vi "sub vi - cycle&temp fail v7.vi"(0 "Amps Lo?":bool, 2 "Input Cluster":T1, 3 "SELECT":T2(ring), 4 "Amps Hi?":bool, 5 "Result In":bool) -> (15 "(FAIL) out":cluster{"FAIL LO":dbl, "FAIL HI":dbl}, 16 "(DISP) out":T3, 17 "T-RISE":cluster{"T-RISE (L)":dbl, "T-RISE (N)":dbl}, 18 "Result Out":bool, 19 "file error":errorcluster)   [LabVIEW 2017]
uses:
  Global display 3.vi
  Global 1.vi
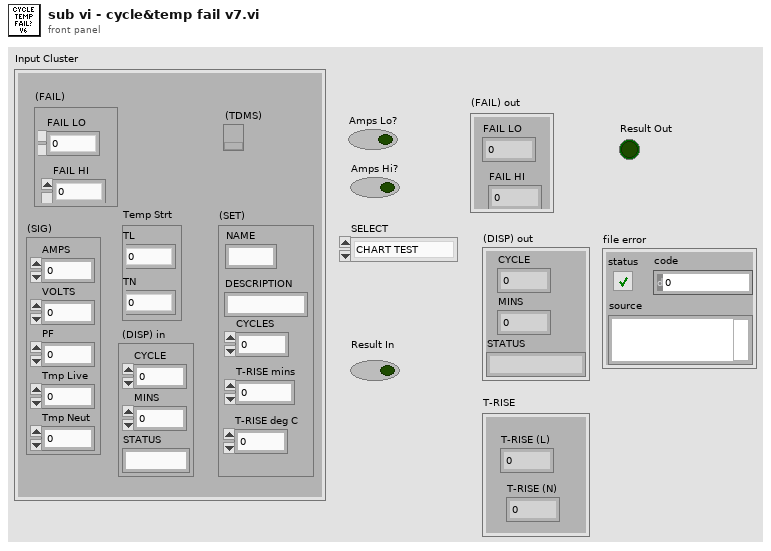
[diagram p1: front panel]
types:
  T1 = cluster{"(FAIL)":cluster{"FAIL LO":dbl, "FAIL HI":dbl}, "(SIG)":cluster{"AMPS":dbl, "VOLTS":dbl, "PF":dbl, "Tmp Live":dbl, "Tmp Neut":dbl}, "Temp Strt":cluster{"TL":dbl, "TN":dbl}, " (DISP) in":cluster{"CYCLE":dbl, "MINS":dbl, "STATUS":string}, "(SET)":cluster{"NAME":string, "DESCRIPTION":string, "CYCLES":dbl, "T-RISE mins":dbl, "T-RISE deg C":dbl}, "(TDMS)":refnum<k34>}
  T2 = enum32{"CHART TEST", "CYCLE TEST", "T-RISE TEST"}
  T3 = cluster{"CYCLE":dbl, "MINS":dbl, "STATUS":string}
  T4 = cluster{"AMPS":dbl, "VOLTS":dbl, "PF":dbl, "Tmp Live":dbl, "Tmp Neut":dbl}
  T5 = cluster{"NAME":string, "DESCRIPTION":string, "CYCLES":dbl, "T-RISE mins":dbl, "T-RISE deg C":dbl}
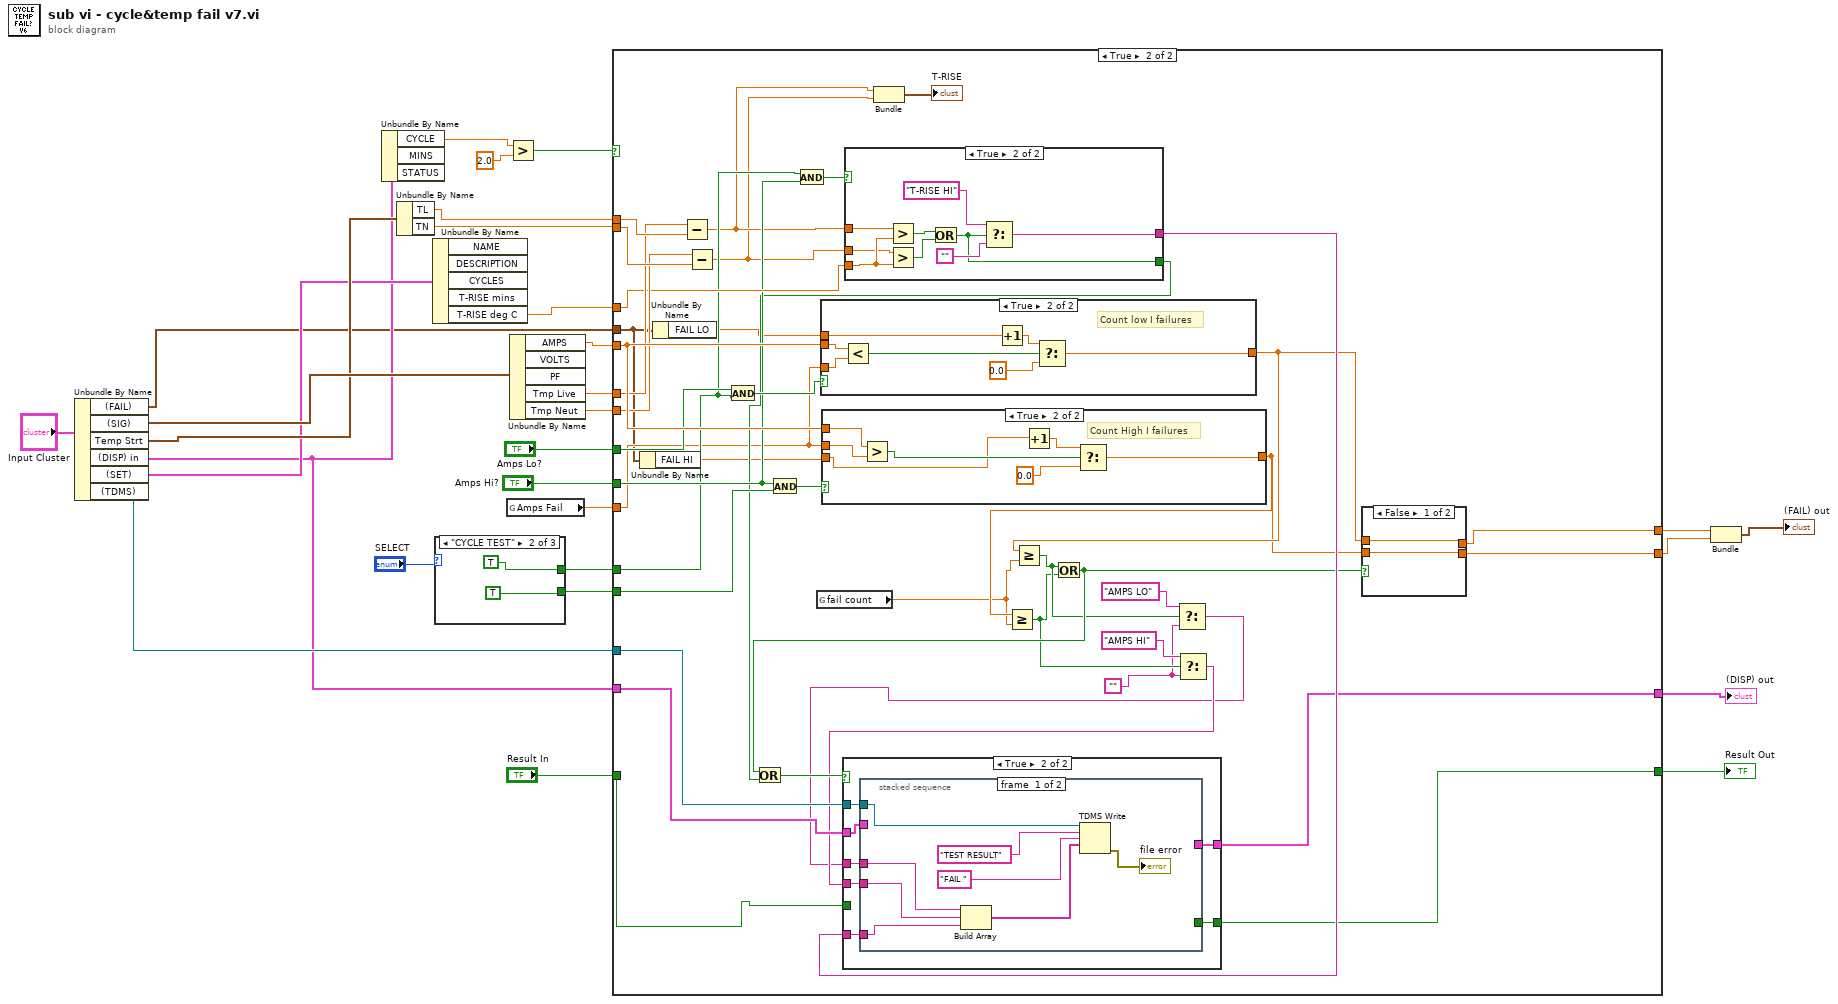
[diagram p0: block diagram]
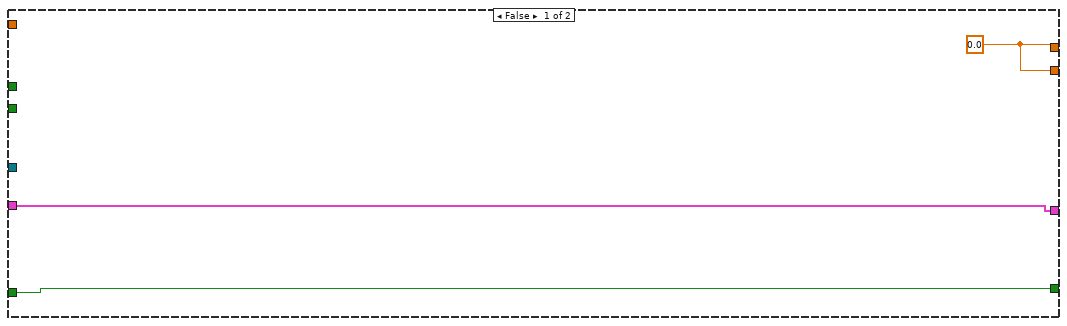
[diagram p2: hidden frame]
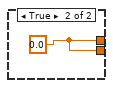
[diagram p3: hidden frame]
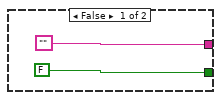
[diagram p4: hidden frame]
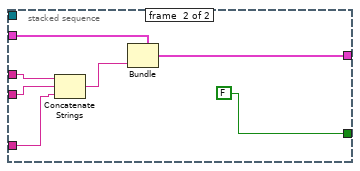
[diagram p6: hidden frame]
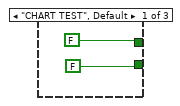
[diagram p9: hidden frame]
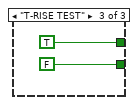
[diagram p10: hidden frame]
diagram:
  n1 = Unbundle By Name("Input Cluster") -> ("(FAIL)"=w1:cluster{"FAIL LO":dbl, "FAIL HI":dbl}, "(SIG)"=w16:T4, "Temp Strt"=w15:cluster{"TL":dbl, "TN":dbl}, "(DISP) in"=w6:T3, "(SET)"=w14:T5, "(TDMS)"=w13:refnum<k34>)
  n2 = Unbundle By Name(w6) -> ("CYCLE"=w5:dbl)  [unwired: 2 out]
  n3 = Unbundle By Name(w15) -> ("TL"=w3:dbl, "TN"=w2:dbl)
  n4 = Unbundle By Name(w14) -> ("T-RISE deg C"=w24:dbl)  [unwired: 4 out]
  n5 = case shown="\"CYCLE TEST\"" "SELECT" {
    tunnel: [FALSE TRUE TRUE] -> w20
    tunnel: [FALSE TRUE FALSE] -> w23
    frame "CHART TEST", Default {
    }
    frame "CYCLE TEST" {
    }
    frame "T-RISE TEST" {
    }
  }
  n6 = global read "Global display 3.vi" "Amps Fail"() -> (w4:dbl)
  n7 = Greater?(x=w5, y=2.0) -> (0:w18:bool)
  n8 = Unbundle By Name(w16) -> ("AMPS"=w27:dbl, "Tmp Live"=w26:dbl, "Tmp Neut"=w25:dbl)  [unwired: 2 out]
  n9 = case shown="True" w18 {
    tunnel: w27 -> [_ w78]
    tunnel: w13 -> [_ w77]
    tunnel: w6 -> [w36 w76]
    tunnel: w3 -> [_ w75]
    tunnel: w2 -> [_ w74]
    tunnel: w26 -> [_ w73]
    tunnel: w25 -> [_ w72]
    tunnel: w24 -> [_ w71]
    tunnel: w23 -> [_ w68]
    tunnel: "Amps Lo?" -> [_ w66]
    tunnel: "Amps Hi?" -> [_ w64]
    tunnel: w20 -> [_ w63]
    tunnel: [w37 w60] -> w11
    tunnel: [w37 w59] -> w10
    tunnel: [w36 w58] -> w9
    tunnel: [w35 w57] -> w8
    tunnel: "Result In" -> [w35 w56]
    tunnel: w4 -> [_ w41]
    tunnel: w1 -> [_ w39]
    frame False {
      w37 = 0.0
    }
    frame True {
      w48 = ""
      n10 = Unbundle By Name(w39) -> ("FAIL HI"=w38:dbl)
      n11 = Unbundle By Name(w39) -> ("FAIL LO"=w40:dbl)
      n12 = Subtract(x=w73, y=w75) -> (x-y=w45:dbl)
      n13 = Subtract(x=w72, y=w74) -> (x-y=w44:dbl)
      n14 = And(x=w66, y=w63) -> (x .and. y?=w67:bool)
      n15 = And(x=w64, y=w68) -> (x .and. y?=w69:bool)
      n16 = And(x=w63, y=w64) -> (x .and. y?=w65:bool)
      n17 = global read "Global 1.vi" "fail count"() -> (w42:dbl)
      n18 = case shown="True" w67 {
        tunnel: w78 -> [_ w132]
        tunnel: w41 -> [_ w131]
        tunnel: w40 -> [w125 w127]
        tunnel: [w125 w126] -> w62
        frame False {
        }
        frame True {
          # "Count low I failures"
          n19 = Less?(x=w132, y=w131) -> (x < y?=w130:bool)
          n20 = Increment(x=w127) -> (x+1=w129:dbl)
          n21 = Select(t=w129, s=w130, f=0.0) -> (s? t:f=w126:dbl)
        }
      }
      n22 = case shown="True" w69 {
        tunnel: w78 -> [_ w124]
        tunnel: w41 -> [_ w123]
        tunnel: [w117 w119] -> w61
        tunnel: w38 -> [w117 w118]
        frame False {
        }
        frame True {
          # "Count High I failures"
          n23 = Greater?(x=w124, y=w123) -> (0:w122:bool)
          n24 = Increment(x=w118) -> (x+1=w121:dbl)
          n25 = Select(t=w121, s=w122, f=0.0) -> (s? t:f=w119:dbl)
        }
      }
      n26 = case shown="True" w65 {
        tunnel: w71 -> [_ w92]
        tunnel: w45 -> [_ w85]
        tunnel: w44 -> [_ w84]
        tunnel: ["" w87] -> w70
        tunnel: [FALSE w86] -> w54
        frame False {
        }
        frame True {
          n27 = Greater?(x=w85, y=w92) -> (0:w90:bool)
          n28 = Greater?(x=w84, y=w92) -> (0:w91:bool)
          n29 = Or(x=w90, y=w91) -> (x .or. y?=w86:bool)
          n30 = Select(t="T-RISE HI", s=w86, f="") -> (s? t:f=w87:string)
        }
      }
      n31 = Bundle(w45, w44) -> (→"T-RISE":cluster{dbl, dbl})  [unwired: 1 in]
      n32 = Greater Or Equal?(x=w61, y=w42) -> (x >= y?=w51:bool)
      n33 = Greater Or Equal?(x=w62, y=w42) -> (x >= y?=w52:bool)
      n34 = Or(x=w52, y=w51) -> (x .or. y?=w55:bool)
      n35 = Or(x=w55, y=w54) -> (x .or. y?=w53:bool)
      n36 = Select(t="AMPS LO", s=w52, f=w48) -> (s? t:f=w46:string)
      n37 = Select(t="AMPS HI", s=w51, f=w48) -> (s? t:f=w47:string)
      n38 = case shown="True" w53 {
        tunnel: w46 -> [_ w101]
        tunnel: w47 -> [_ w100]
        tunnel: w76 -> [w94 w99]
        tunnel: w77 -> [_ w98]
        tunnel: w70 -> [_ w97]
        tunnel: [w94 w96] -> w58
        tunnel: [w93 w95] -> w57
        tunnel: w56 -> [w93 _]
        frame False {
        }
        frame True {
          n39 = stacked-sequence {
            tunnel: w101 -> [w102 w116]
            tunnel: w100 -> [w103 w115]
            tunnel: w99 -> [_ w113]
            tunnel: w98 -> [w105 _]
            tunnel: w97 -> [w104 w112]
            tunnel: [_ w111] -> w96
            tunnel: [_ FALSE] -> w95
            frame #0 {
              n40 = Build Array(w102, w103, w104) -> (w108:string[])
              n41 = TDMS Write(0:w105, 5:"TEST RESULT", 7:"FAIL ", 9:w108) -> (15:→"file error":errorcluster)  [unwired: 2 in, 3 out]
            }
            frame #1 {
              n42 = Concatenate Strings(w116, w115, w112) -> (w114:string)
              n43 = Bundle(cluster=w113, "STATUS"=w114) -> (w111:T3)  [unwired: 2 in]
            }
          }
        }
      }
      n44 = case shown="False" w55 {
        tunnel: w62 -> [w80 _]
        tunnel: w61 -> [w79 _]
        tunnel: [w80 w81] -> w60
        tunnel: [w79 w81] -> w59
        frame False {
        }
        frame True {
          w81 = 0.0
        }
      }
    }
  }
  "(DISP) out" <- w9
  "Result Out" <- w8
  n45 = Bundle("FAIL LO"=w11, "FAIL HI"=w10) -> (→"(FAIL) out":cluster{"FAIL LO":dbl, "FAIL HI":dbl})  [unwired: 1 in]
